vi "Write # tantrums thrown.vi"(8 "error in (no error)":errorcluster, 10 "# tantrums thrown":i32, 11 "Tiger Woods in":refnum<class "Tiger Woods.lvclass">) -> (0 "error out":errorcluster, 3 "Tiger Woods out":refnum<class "Tiger Woods.lvclass">)   [LabVIEW 2019, in "Tiger Woods.lvclass"]
uses:
  Tiger Woods.lvclass
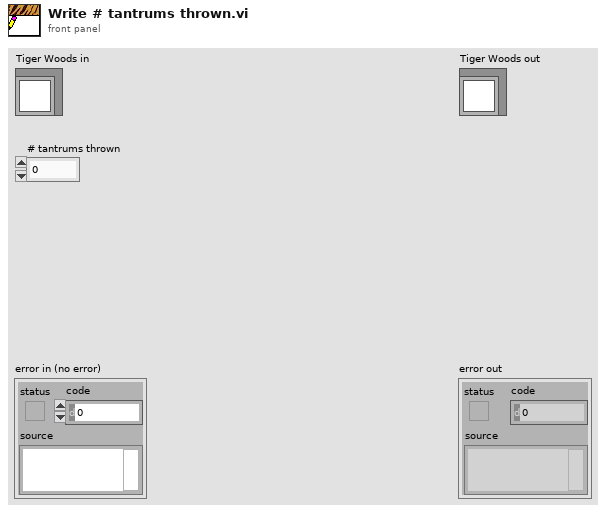
[diagram p1: front panel]
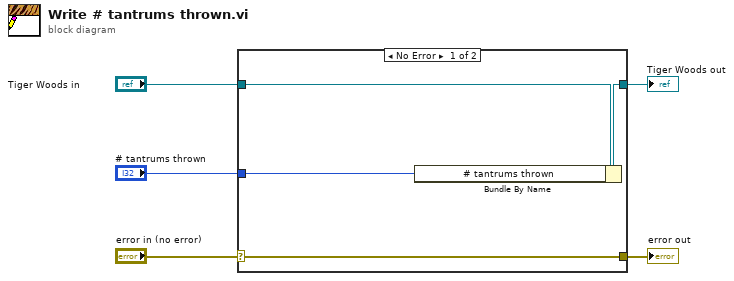
[diagram p0: block diagram]
diagram:
  n1 = case shown="No Error" "error in (no error)" {
    selector: "error in (no error)" -> [w9 w10]
    tunnel: [w9 w10] -> w4
    tunnel: [w7 w11] -> w2
    tunnel: "Tiger Woods in" -> [w8 w11]
    tunnel: "# tantrums thrown" -> [w6 _]
    frame No Error {
      n2 = Bundle By Name(cluster=w8, "# tantrums thrown"=w6) -> (w7:refnum<class "Tiger Woods.lvclass">)
    }
    frame Error {
    }
  }
  "error out" <- w4
  "Tiger Woods out" <- w2
